vi "Read Result Wrapper - Reentrant.vi"(8 "error in (no error)":errorcluster, 11 "SimpleArithmetic in":refnum<class "SimpleArithmetic - Reentrant.lvclass">) -> (0 "error out":errorcluster, 2 "Result":dbl, 3 "SimpleArithmetic out":refnum<class "SimpleArithmetic - Reentrant.lvclass">)   [LabVIEW 2010]
uses:
  SimpleArithmetic - Reentrant.lvclass
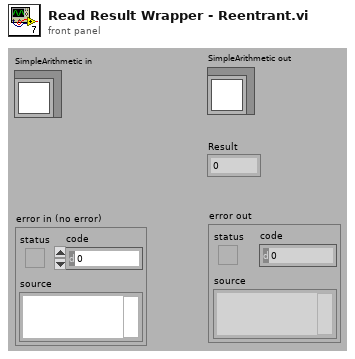
[diagram p1: front panel]
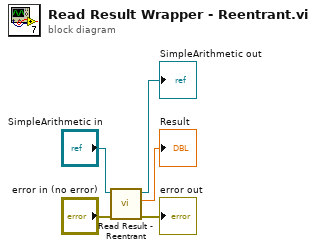
[diagram p0: block diagram]
diagram:
  n1 = call "Read Result - Reentrant.vi"("error in (no error)"="error in (no error)", "SimpleArithmetic in"="SimpleArithmetic in") -> ("error out"=→"error out":errorcluster, "Result"=→"Result":dbl, "SimpleArithmetic out"=→"SimpleArithmetic out":refnum<class "SimpleArithmetic - Reentrant.lvclass">)  [unwired: 7 in]
